vi "HumanTimEtch.vi"(8 "RunCluster":T1, 9 "queue in 2":refnum<queue>, 10 "StepParameters":T5, 11 ".NET Refnum in":refnum<k24>) -> ()   [LabVIEW 2020]
uses:
  D:/PumpAutomation2/DEMPBot2/PumpAdapter.exe
  PumpAdapter.exe
  RunControlCluster.ctl
  MessageQueues.ctl
  <vilib>/httpClient/ClientHandle.ctl
  UserCommands.ctl
  FrontPanelReferences.ctl
  EquipmentDefinition32_1.ctl
  <vilib>/httpClient/LabVIEWHTTPClient.lvlib
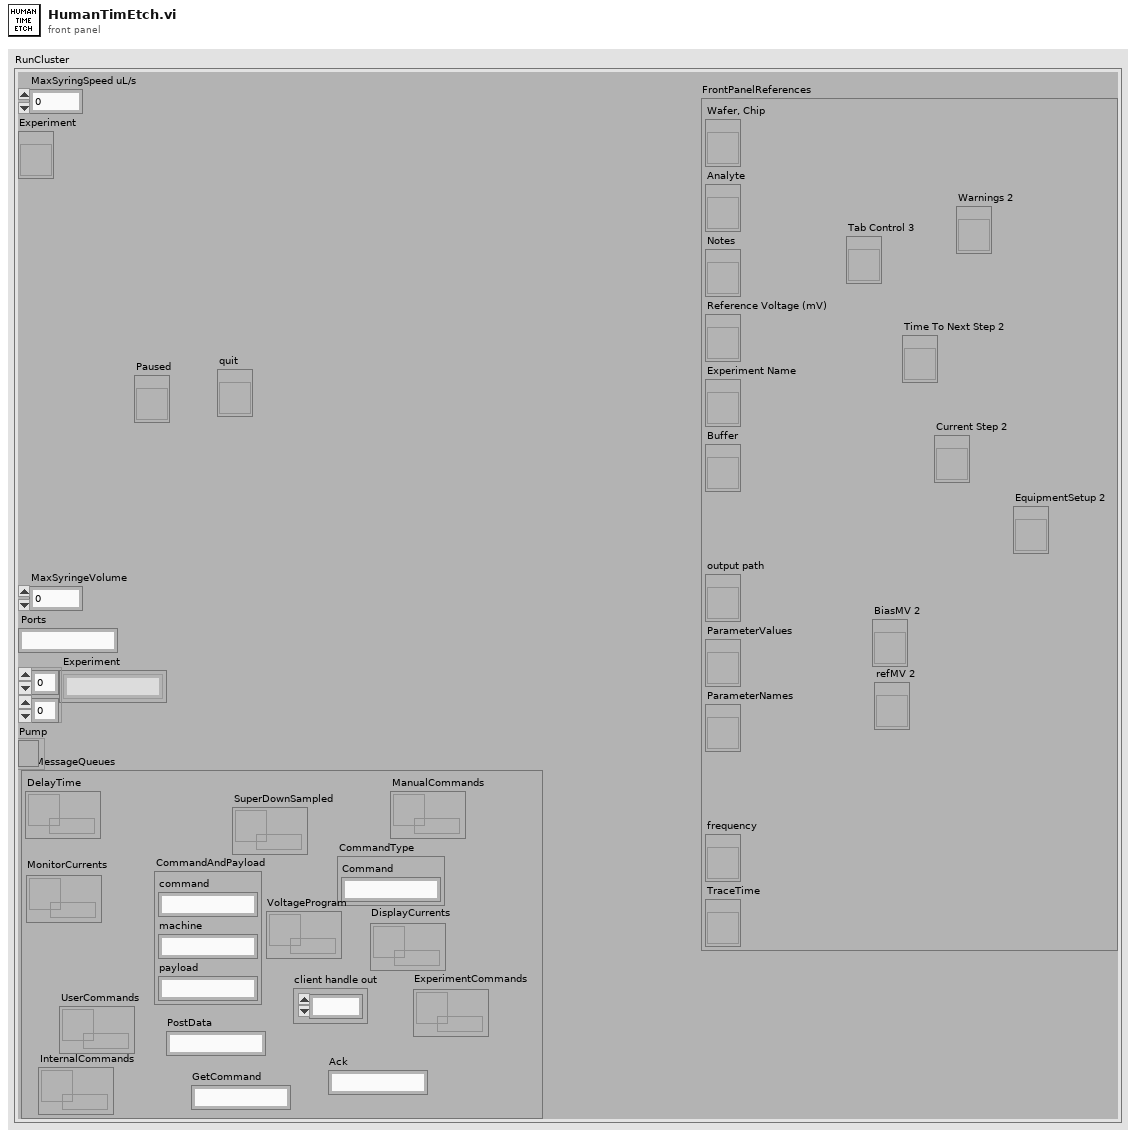
[diagram p1: front panel]
types:
  T1 = typedef "RunControlCluster.ctl" = cluster{"MaxSyringSpeed uL/s":dbl, "Experiment":refnum<vi>, "Paused":refnum<vi>, "MaxSyringeVolume":dbl, "Ports":string, "Experiment":string[][], "Pump":refnum<k24>, "MessageQueues":T2, "quit":refnum<vi>, "FrontPanelReferences":T4}
  T2 = typedef "MessageQueues.ctl" = cluster{"CommandType":cluster{"Command":string}, "CommandAndPayload":cluster{"command":string, "machine":string, "payload":string}, "client handle out":T3, "PostData":string, "GetCommand":string, "Ack":string, "VoltageProgram":refnum<queue>, "ExperimentCommands":refnum<queue>, "DisplayCurrents":refnum<queue>, "MonitorCurrents":refnum<queue>, "InternalCommands":refnum<queue>, "SuperDownSampled":refnum<queue>, "UserCommands":refnum<queue>, "DelayTime":refnum<queue>, "ManualCommands":refnum<queue>}
  T3 = typedef "LabVIEWHTTPClient.lvlib/ClientHandle.ctl" = refnum<k1>
  T4 = typedef "FrontPanelReferences.ctl" = cluster{"Wafer, Chip":refnum<vi>, "Analyte":refnum<vi>, "Notes":refnum<vi>, "Reference Voltage (mV)":refnum<vi>, "Experiment Name":refnum<vi>, "Buffer":refnum<vi>, "output path":refnum<vi>, "ParameterValues":refnum<vi>, "ParameterNames":refnum<vi>, "frequency":refnum<vi>, "TraceTime":refnum<vi>, "Warnings 2":refnum<vi>, "Time To Next Step 2":refnum<vi>, "Current Step 2":refnum<vi>, "Tab Control 3":refnum<vi>, "BiasMV 2":refnum<vi>, "refMV 2":refnum<vi>, "EquipmentSetup 2":refnum<vi>}
  T5 = cluster{"Step":string, "Push":string, "Analyte1":string, "Volume1":dbl, "Analyte2":string, "Measurement":string, "Volume2":dbl, "Speed1":dbl, "Speed2":dbl, "MinTime":dbl, "Bias":dbl, "Slew":dbl, "Parameter1":string, "Parameter2":string}
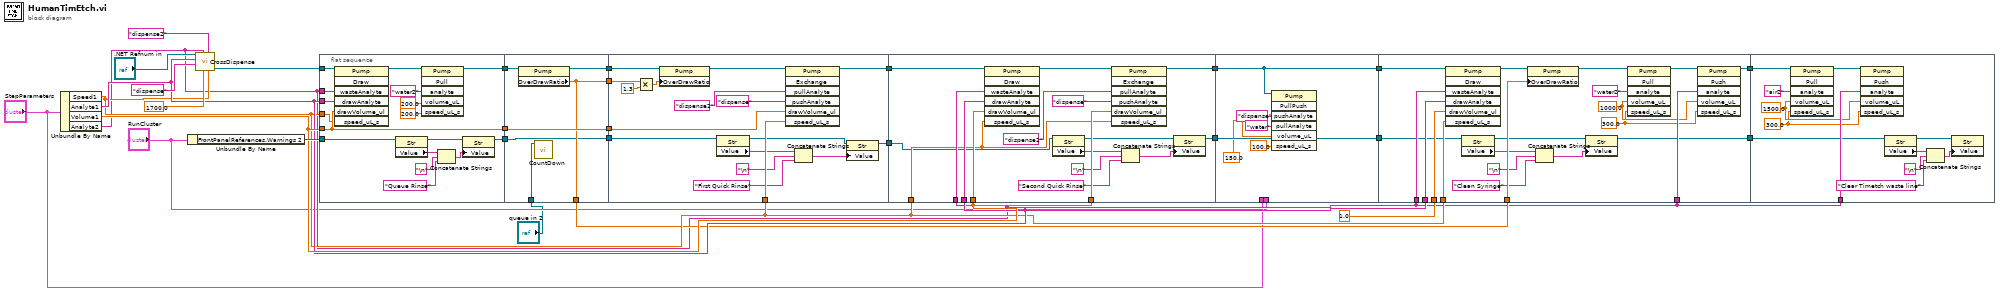
[diagram p0: block diagram]
diagram:
  n1 = Unbundle By Name("StepParameters") -> ("Speed1"=w15:dbl, "Analyte1"=w17:string, "Volume1"=w19:dbl, "Analyte2"=w13:string)
  n2 = Unbundle By Name("RunCluster") -> ("FrontPanelReferences.Warnings 2"=w22:refnum<vi>)
  n3 = call "CrossDispense.vi"("speed_uL_s"=w15, "wasteLine"="dispense2" ("wasteAnalyte"), "drawVolume_ul"=1700.0, "airWaste2"=w13, "dispenseLine"="dispense", "drawAnalyte"=w17, "Pump in"=".NET Refnum in") -> ("Pump out"=w25:refnum<k24>)  [unwired: 3 in, 1 out]
  n4 = flat-sequence {
    tunnel: w25 -> [w47]
    tunnel: w17 -> [w46]
    tunnel: w13 -> [w45]
    tunnel: w19 -> [w43]
    tunnel: [w34] -> w10
    tunnel: [w43] -> w9
    tunnel: w15 -> [w42]
    tunnel: w22 -> [w36]
    tunnel: [w35] -> w8
    tunnel: w10 -> [w52]
    tunnel: [w51] -> w30
    tunnel: w9 -> [w53]
    tunnel: [w53] -> w29
    tunnel: [w50] -> w14
    tunnel: [w50] -> w23
    tunnel: w8 -> [w49]
    tunnel: [w49] -> w21
    tunnel: "queue in 2" -> [w48]
    tunnel: w30 -> [w70]
    tunnel: w29 -> [w69]
    tunnel: w15 -> [w68]
    tunnel: w23 -> [w61]
    tunnel: w21 -> [w55]
    tunnel: [w65] -> w20
    tunnel: [w54] -> w18
    tunnel: w20 -> [w83]
    tunnel: w19 -> [w84]
    tunnel: w13 -> [w82]
    tunnel: w17 -> [w81]
    tunnel: w19 -> [w80]
    tunnel: w15 -> [w79]
    tunnel: w18 -> [w72]
    tunnel: [w78] -> w7
    tunnel: [w71] -> w5
    tunnel: w7 -> [w92]
    tunnel: [w92] -> w6
    tunnel: w5 -> [w93]
    tunnel: [w93] -> w4
    tunnel: "StepParameters" -> [_]
    tunnel: "RunCluster" -> [_]
    tunnel: w6 -> [w107]
    tunnel: w13 -> [w111]
    tunnel: w13 -> [w106]
    tunnel: w17 -> [w105]
    tunnel: 1.0 ("drawVolume_ul") -> [w104]
    tunnel: w15 -> [w103]
    tunnel: w14 -> [w102]
    tunnel: w4 -> [w96]
    tunnel: [w95] -> w12
    tunnel: [w94] -> w11
    tunnel: w13 -> [w125]
    tunnel: w12 -> [w122]
    tunnel: w11 -> [w115]
    frame #0 {
      n5 = invoke class="Pump" method="Draw"(reference=w47, "wasteAnalyte"=w45, "drawAnalyte"=w46, "drawVolume_ul"=w43, "speed_uL_s"=w42) -> (reference out=w44:refnum<k24>)  [unwired: 2 in, 6 out]
      n6 = property class="Str"(reference=w36) -> (reference out=w41:refnum<vi>, "Value"=w40:string)  [unwired: 1 in, 1 out]
      n7 = invoke class="Pump" method="Pull"(reference=w44, "analyte"="water2", "volume_uL"=200.0, "speed_uL_s"=200.0) -> (reference out=w34:refnum<k24>)  [unwired: 2 in, 5 out]
      n8 = Concatenate Strings(w40, "\n" ("string"), "Queue Rinse" ("string")) -> (w37:string)
      n9 = property class="Str"(reference=w41, "Value"=w37) -> (reference out=w35:refnum<vi>)  [unwired: 1 in, 1 out]
    }
    frame #1 {
      n10 = property class="Pump"(reference=w52) -> (reference out=w51:refnum<k24>, "OverDrawRatio"=w50:dbl)  [unwired: 1 in, 1 out]
      n11 = call "CountDown.vi"("queue in 2"=w48) -> ()  [unwired: 11 in]
    }
    frame #2 {
      n12 = Multiply(x=w61, y=1.3 ("OverDrawRatio")) -> (x*y=w62:dbl)
      n13 = property class="Pump"(reference=w70, "OverDrawRatio"=w62) -> (reference out=w64:refnum<k24>)  [unwired: 1 in, 1 out]
      n14 = property class="Str"(reference=w55) -> (reference out=w60:refnum<vi>, "Value"=w59:string)  [unwired: 1 in, 1 out]
      n15 = invoke class="Pump" method="Exchange"(reference=w64, "pullAnalyte"="dispense2", "pushAnalyte"="dispense", "drawVolume_ul"=w69, "speed_uL_s"=w68) -> (reference out=w65:refnum<k24>)  [unwired: 2 in, 6 out]
      n16 = Concatenate Strings(w59, "\n" ("string"), "First Quick Rinse" ("string")) -> (w56:string)
      n17 = property class="Str"(reference=w60, "Value"=w56) -> (reference out=w54:refnum<vi>)  [unwired: 1 in, 1 out]
    }
    frame #3 {
      n18 = invoke class="Pump" method="Draw"(reference=w83, "wasteAnalyte"=w82, "drawAnalyte"=w81, "drawVolume_ul"=w80, "speed_uL_s"=w79) -> (reference out=w87:refnum<k24>)  [unwired: 2 in, 6 out]
      n19 = property class="Str"(reference=w72) -> (reference out=w77:refnum<vi>, "Value"=w76:string)  [unwired: 1 in, 1 out]
      n20 = invoke class="Pump" method="Exchange"(reference=w87, "pullAnalyte"="dispense2", "pushAnalyte"="dispense", "drawVolume_ul"=w84, "speed_uL_s"=w79) -> (reference out=w78:refnum<k24>)  [unwired: 2 in, 6 out]
      n21 = Concatenate Strings(w76, "\n" ("string"), "Second Quick Rinse" ("string")) -> (w73:string)
      n22 = property class="Str"(reference=w77, "Value"=w73) -> (reference out=w71:refnum<vi>)  [unwired: 1 in, 1 out]
    }
    frame #4 {
      n23 = invoke class="Pump" method="PullPush"(reference=w92, "pushAnalyte"="dispense", "pullAnalyte"="water", "volume_uL"=150.0 ("Volume1"), "speed_uL_s"=100.0) -> ()  [unwired: 2 in, 7 out]
    }
    frame #5 {
      w109 = 300.0 ("speed_uL_s")
      w110 = 1000.0 ("volume_uL")
      n24 = invoke class="Pump" method="Draw"(reference=w107, "wasteAnalyte"=w106, "drawAnalyte"=w105, "drawVolume_ul"=w104, "speed_uL_s"=w103) -> (reference out=w112:refnum<k24>)  [unwired: 2 in, 6 out]
      n25 = property class="Str"(reference=w96) -> (reference out=w101:refnum<vi>, "Value"=w100:string)  [unwired: 1 in, 1 out]
      n26 = property class="Pump"(reference=w112, "OverDrawRatio"=w102) -> (reference out=w113:refnum<k24>)  [unwired: 1 in, 1 out]
      n27 = Concatenate Strings(w100, "\n" ("string"), "Clean Syringe" ("string")) -> (w97:string)
      n28 = property class="Str"(reference=w101, "Value"=w97) -> (reference out=w94:refnum<vi>)  [unwired: 1 in, 1 out]
      n29 = invoke class="Pump" method="Pull"(reference=w113, "analyte"="water2", "volume_uL"=w110, "speed_uL_s"=w109) -> (reference out=w114:refnum<k24>)  [unwired: 2 in, 5 out]
      n30 = invoke class="Pump" method="Push"(reference=w114, "analyte"=w111, "volume_uL"=w110, "speed_uL_s"=w109) -> (reference out=w95:refnum<k24>)  [unwired: 2 in, 5 out]
    }
    frame #6 {
      w123 = 300.0 ("speed_uL_s")
      w124 = 1500.0 ("volume_uL")
      n31 = invoke class="Pump" method="Pull"(reference=w122, "analyte"="air2", "volume_uL"=w124, "speed_uL_s"=w123) -> (reference out=w126:refnum<k24>)  [unwired: 2 in, 5 out]
      n32 = invoke class="Pump" method="Push"(reference=w126, "analyte"=w125, "volume_uL"=w124, "speed_uL_s"=w123) -> ()  [unwired: 2 in, 6 out]
      n33 = property class="Str"(reference=w115) -> (reference out=w120:refnum<vi>, "Value"=w119:string)  [unwired: 1 in, 1 out]
      n34 = Concatenate Strings(w119, "\n" ("string"), "Clear Timetch waste line" ("string")) -> (w117:string)
      n35 = property class="Str"(reference=w120, "Value"=w117) -> ()  [unwired: 1 in, 2 out]
    }
  }
